vi "FPGA Based CAN decoding.vi"() -> ()   [LabVIEW 2016]
doc: "This example transmits one frame contained in Data Frame every time the Write button is pressed. After building this FPGA VI, you run it using CAN Channel Transmit (Host).vi (not standalone).\n\nThis example assumes the following configuration for CAN 0: Auto Start = True, Listen Only = False, Input Timeout = 10000ms, Output Timeout = 10000ms. The CAN Output node is configured to use an array of U32 for the CAN frame. For more information on configuration, refer to the Help for the NI 9853 CAN module."
uses:
  <vilib>/rvi/Emulation/niFpgaCriticalErrorInLSC.vi
  <vilib>/rvi/eio/common/nirviEmuTemplateMethod_errors.vi
  <vilib>/rvi/Emulation/niFpgaEmulationReportErrorSimple.vi
  <vilib>/rvi/Emulation/niFpgaSctlEmulationGetInTimedLoop.vi
  <vilib>/rvi/Emulation/niFpgaGetClockAttributes.vi
  <vilib>/rvi/Emulation/niFpgaProcessEmulError.vi
  <vilib>/LabVIEW Targets/FPGA/RIO/nicrio_985x_controls.llb/CAN_IO_Frame Cluster.ctl
  <vilib>/LabVIEW Targets/FPGA/RIO/nicrio_985x_controls.llb/CAN_IO_Frame Type.ctl
  <vilib>/eio/EIONode/EIONode.xnode
  <vilib>/eio/EIOMethodNode/EIOMethodNode.xnode
  <vilib>/rvi/DataTransferAndStorage/Container/XNode/niFpgaContainer.xnode
  <vilib>/LabVIEW Targets/FPGA/RIO/nicrio_985x_controls.llb/CAN_IO_Frame Array U32.ctl
  <vilib>/rvi/FIFO/Fifo_Resource/nirvififoEmulationRead.vi
  <vilib>/rvi/FIFO/Fifo_Resource/nirvififoEmulationWrite.vi
  <vilib>/rvi/FIFO/Fifo_Resource/nirvififoEmulationClear.vi
panel:
  out "Motor power":u8
  out "Ready to drive":bool
  out "cooling liquid temperature":u8
  out "accelerator position":u8
  out "brake pedal position":u8
  out "CAN Frame Out":T1 {"Data" format="%.0x"; "DataLength" format="%.0x"; "InfoB" format="%.0x"; "InfoA" format="%.0x"; "Type" format="%.0x"; "Identifier" format="%.0x"; "Timestamp" format="%.0x"}
  in  "CAN Frame In":T1={"Timestamp"=0, "Identifier"=0, "Type"=0, "InfoA"=0, "InfoB"=0, "DataLength"=0, "Data"=[0, 0, 0, 0, 0, 0, 0, 0]} {"Data" format="%.0x"; "DataLength" format="%.0x"; "InfoB" format="%.0x"; "InfoA" format="%.0x"; "Type" format="%.0x"; "Identifier" format="%.0x"; "Timestamp" format="%.0x"}
  out "FIFO Full":bool
  in  "Write":bool
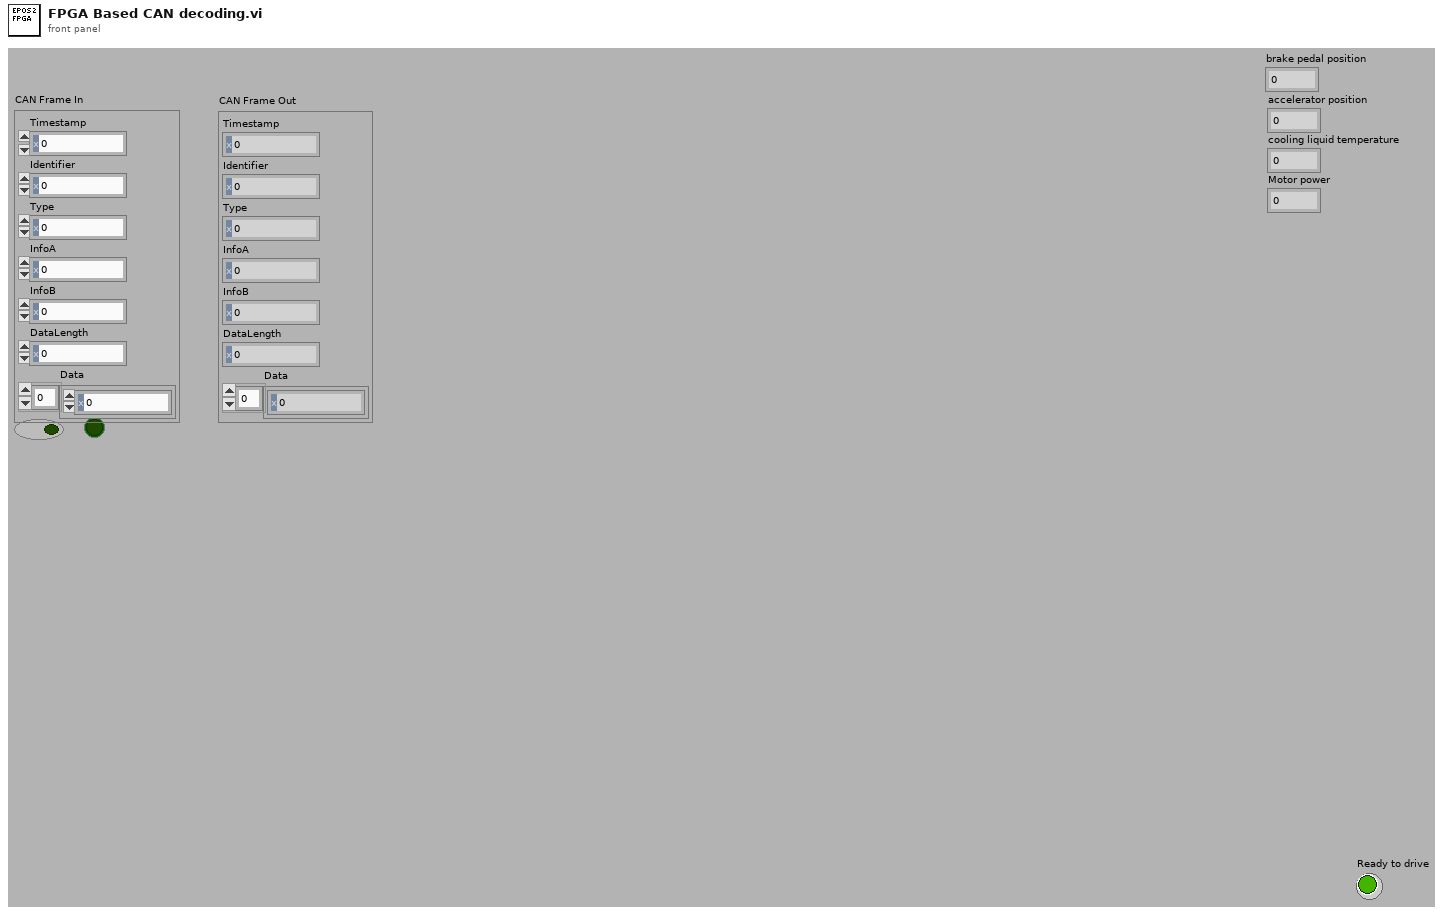
[diagram p1: front panel]
types:
  T1 = cluster{"Timestamp":u64, "Identifier":u32, "Type":u8, "InfoA":u8, "InfoB":u8, "DataLength":u8, "Data":u8[]}
  T2 = typedef "CAN_IO_Frame Cluster.ctl" = cluster{"timestamp high":u32, "timestamp low":u32, "identifier":u32, "type":T3, "info A":u8, "info B":u8, "data length":u8, "data":u8[]}
  T3 = typedef "CAN_IO_Frame Type.ctl" = enum8{"Data Frame", "Remote Frame", "(reserved)", "(reserved) ", "(reserved)  ", "(reserved)   ", "Bus Error", "Transceiver Fault"}
  T4 = cluster{"data[0]":u8, "data[1]":u8, "data[2]":u8, "data[3]":u8, "data[4]":u8, "data[5]":u8, "data[6]":u8, "data[7]":u8, "data[8]":u8}
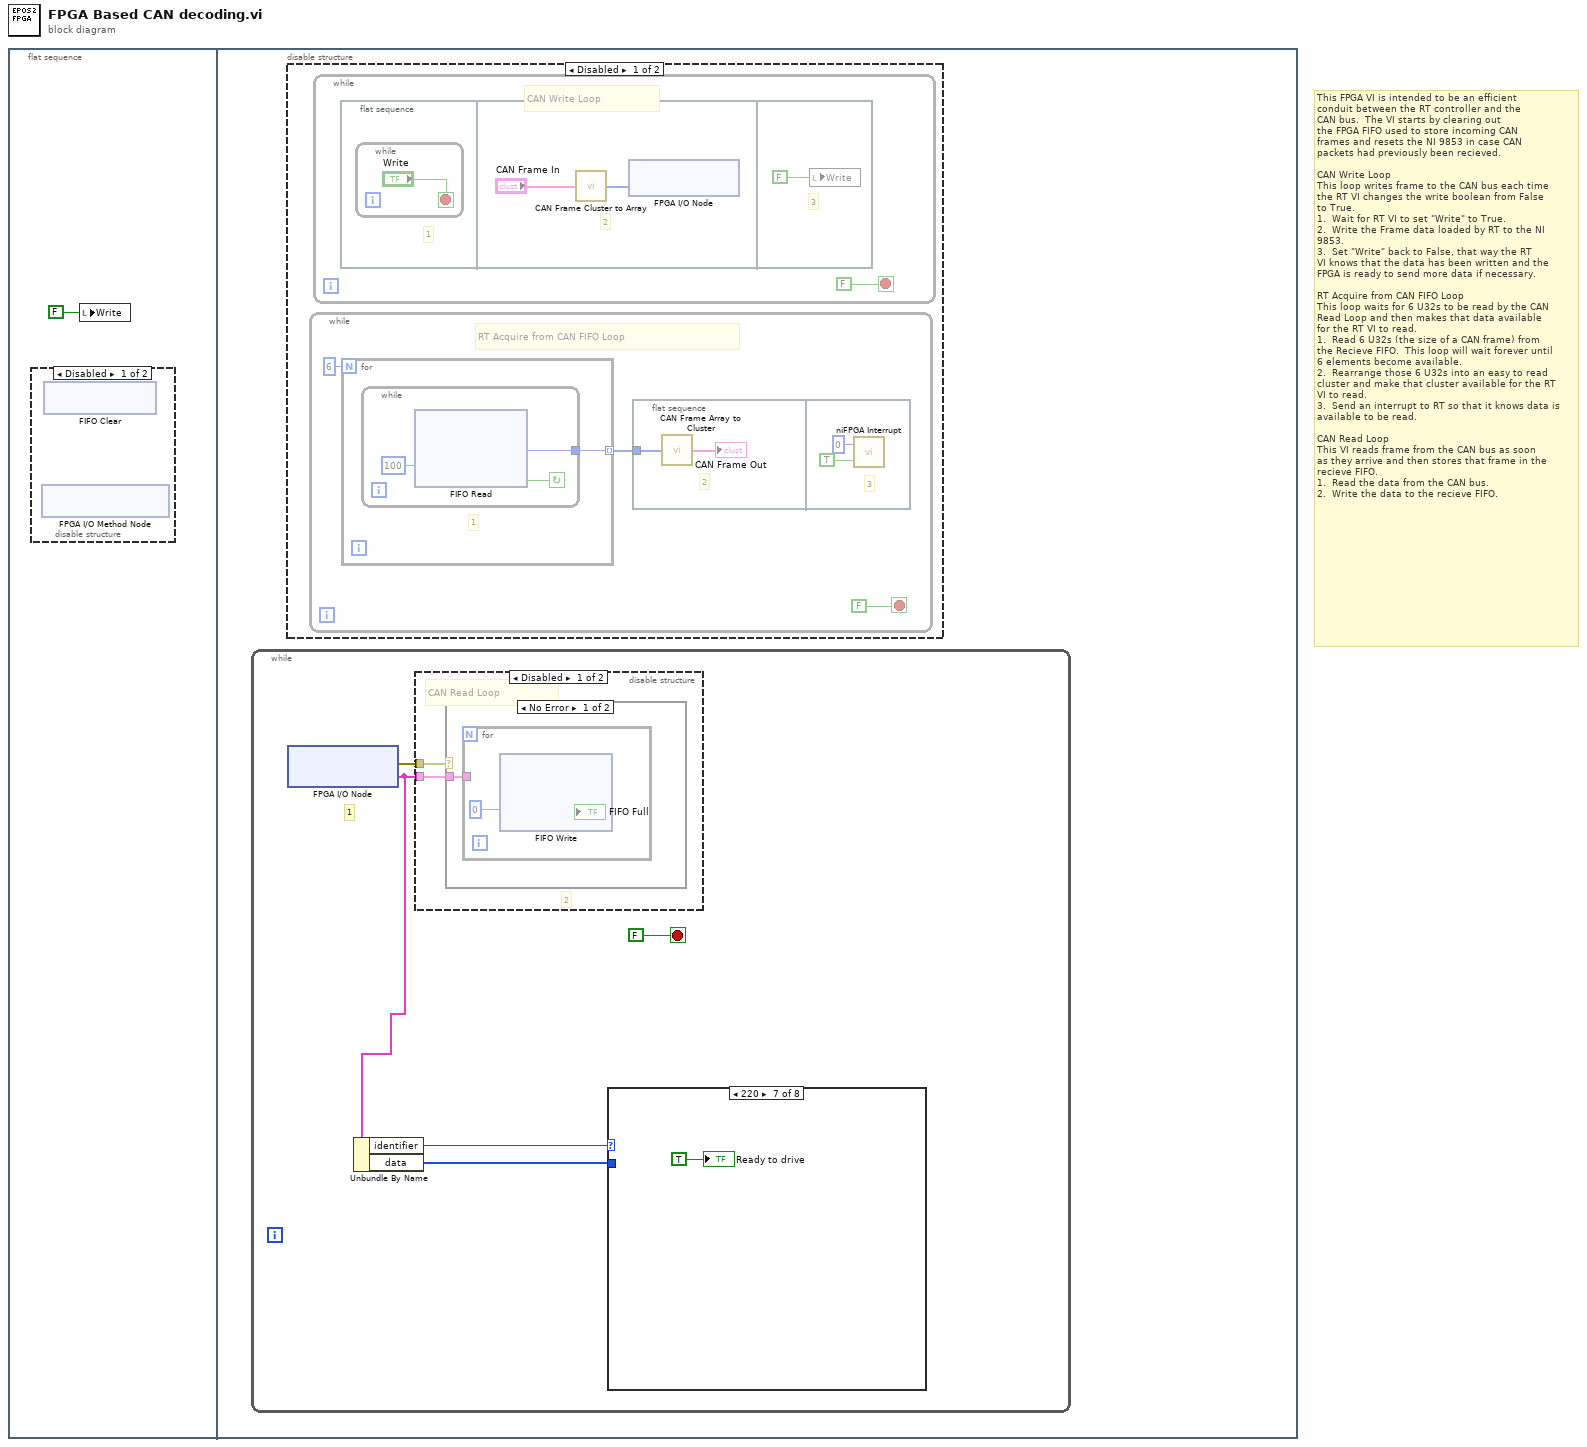
[diagram p0: block diagram]
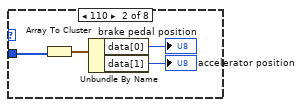
[diagram p7: hidden frame]
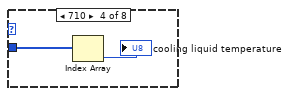
[diagram p9: hidden frame]
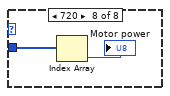
[diagram p12: hidden frame]
diagram:
  # "This FPGA VI is intended to be an efficient\nconduit between the RT controller and the\nCAN bus.  The VI starts by clearing out\nthe FPGA FIFO used to store incoming CAN\nframes and resets the NI 9853 in case CAN\npackets had previously been recieved.\n\nCAN Write Loop\nThis loop writes frame to the CAN bus each time\nthe RT VI changes the write boolean from False\nto True.\n1.  Wait for RT VI to set \"Write\" to True.\n2.  Write the Frame data loaded by RT to the NI\n9853.\n3.  Set \"Write\" back to False, that way the RT\nVI knows that the data has been written and the\nFPGA is ready to send more data if necessary.\n\nRT Acquire from CAN FIFO Loop\nThis loop waits for 6 U32s to be read by the CAN\nRead Loop and then makes that data available\nfor the RT VI to read.\n1.  Read 6 U32s (the size of a CAN frame) from\nthe Recieve FIFO.  This loop will wait forever until\n6 elements become available.\n2.  Rearrange those 6 U32s into an easy to read\ncluster and make that cluster available for the RT\nVI to read.\n3.  Send an interrupt to RT so that it knows data is\navailable to be read.\n\nCAN Read Loop\nThis VI reads frame from the CAN bus as soon\nas they arrive and then stores that frame in the\nrecieve FIFO.\n1.  Read the data from the CAN bus.\n2.  Write the data to the recieve FIFO."
  n1 = flat-sequence {
    frame #0 {
      n2 = disable-structure shown="Disabled" {
        frame Disabled {
          n3 = xnode "FPGA I/O Method Node"() -> ()  [unwired: 1 in, 1 out]
          n4 = xnode ("FIFO Clear")() -> ()  [unwired: 1 in, 1 out]
        }
        frame Enabled {
        }
      }
      n5 = local write "Write"(FALSE) -> ()
    }
    frame #1 {
      n6 = while {
        stop <- FALSE stop-if-true
        # "1"
        n7 = xnode "FPGA I/O Node"() -> ("error out"=w21:errorcluster, "Mod1/CAN1"=w20:T2)  [unwired: 2 in, 1 out]
        n8 = Unbundle By Name(w20) -> ("identifier"=w19:u32, "data"=w18:u8[])
        n9 = disable-structure shown="Disabled" {
          disable-tunnel: w21 -> [w24 _]
          disable-tunnel: w20 -> [w23 _]
          frame Disabled {
            # "2"
            # "CAN Read Loop"
            n10 = case shown="No Error" w24 {
              tunnel: w23 -> [w25 _]
              frame No Error {
                n11 = for {
                  tunnel: w25 -> [_]
                  n12 = xnode ("FIFO Write")("Timeout"=0) -> ("Timed Out?"=→"FIFO Full":bool)  [unwired: 2 in, 1 out]
                }
              }
              frame Error {
              }
            }
          }
          frame Enabled {
          }
        }
        n13 = case shown="220" w19 {
          tunnel: w18 -> [_ w31 _ w33 _ _ _ w36]
          frame Default {
          }
          frame 110 {
            n14 = Array To Cluster(array=w31) -> (cluster=w30:T4)
            n15 = Unbundle By Name(w30) -> ("data[0]"=→"brake pedal position":u8, "data[1]"=→"accelerator position":u8)
          }
          frame 10 {
          }
          frame 710 {
            n16 = Index Array(array=w33) -> (element=→"cooling liquid temperature":u8)  [unwired: 1 in]
          }
          frame 90 {
          }
          frame 120 {
          }
          frame 220 {
            "Ready to drive" <- TRUE ("Ready to drive")
          }
          frame 720 {
            n17 = Index Array(array=w36) -> (element=→"Motor power":u8)  [unwired: 1 in]
          }
        }
      }
      n18 = disable-structure shown="Disabled" {
        frame Disabled {
          n19 = while {
            stop <- FALSE stop-if-true
            # "RT Acquire from CAN FIFO Loop"
            n20 = for {
              N: 6 -> [_]
              tunnel: [w9] -> w2 mode=indexing
              # "1"
              n21 = while {
                tunnel: [w10] -> w9
                stop <- w11 continue-if-true
                n22 = xnode ("FIFO Read")("Timeout"=100 ("Timeout (-1 for no timeout)")) -> ("Element"=w10:u32, "Timed Out?"=w11:bool)  [unwired: 1 in, 1 out]
              }
            }
            n23 = flat-sequence {
              tunnel: w2 -> [w6]
              frame #0 {
                # "2"
                n24 = call "CAN Frame Array to Cluster.vi"("CAN Frame Array In"=w6) -> ("CAN Frame Cluster Out"=→"CAN Frame Out":T1)
              }
              frame #1 {
                # "3"
                n25 = call <vilib>:"niFPGA Interrupt.vi"("Wait Until Cleared (F)"=TRUE ("Wait Until Cleared"), "IRQ Number (0)"=u8 0 ("IRQ Number")) -> ()  [unwired: 1 in]
              }
            }
          }
          n26 = while {
            stop <- FALSE stop-if-true
            # "CAN Write Loop"
            n27 = flat-sequence {
              frame #0 {
                # "1"
                n28 = while {
                  stop <- "Write" stop-if-true
                }
              }
              frame #1 {
                # "2"
                n29 = call "CAN Frame Cluster to Array.vi"("CAN Frame Cluster In"="CAN Frame In") -> ("CAN Frame Array Out"=w16:u32[])
                n30 = xnode "FPGA I/O Node"("Mod1/CAN1"=w16) -> ()  [unwired: 1 in, 1 out]
              }
              frame #2 {
                # "3"
                n31 = local write "Write"(FALSE ("Write")) -> ()
              }
            }
          }
        }
        frame Enabled {
        }
      }
    }
  }
